vi "getInheritanceChain.vi"(8 "error in (no error)":errorcluster, 11 "Graph in":refnum<class "Graph.lvclass">) -> (0 "error out":errorcluster, 2 "Inheritance Chain":string[](array[string]), 3 "Graph out":refnum<class "Graph.lvclass">)   [LabVIEW 2009, in "Graph.lvclass"]
doc: "Returns the inheritance chain."
uses:
  Graph.lvclass
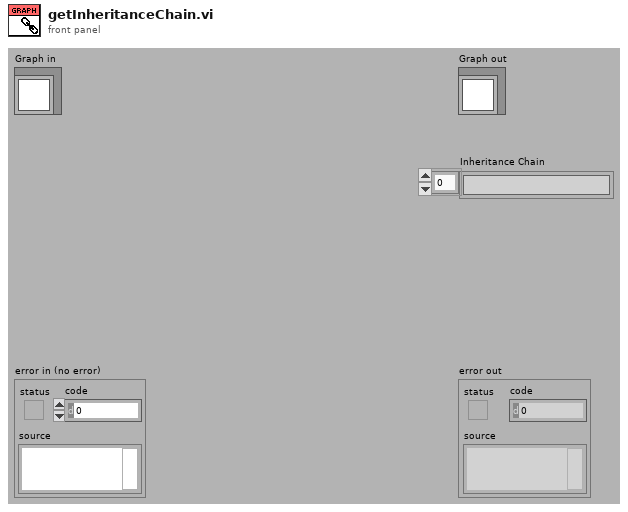
[diagram p1: front panel]
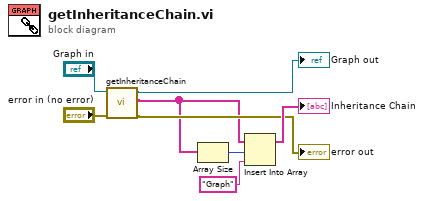
[diagram p0: block diagram]
diagram:
  n1 = call-parent "getInheritanceChain.vi"("error in (no error)"="error in (no error)", "Structure in"="Graph in") -> ("error out"=→"error out":errorcluster, "Inheritance Chain"=w1:string[], "Structure out"=→"Graph out":refnum<class "Graph.lvclass">)  [unwired: 7 in]
  n2 = Array Size(array=w1) -> (size(s)=w6:i32)
  n3 = Insert Into Array(array=w1, index=w6, new element="Graph") -> (→"Inheritance Chain":string[])
